vi "Dialog Box - One Button.vi"(4 "Display On Error (True)":bool=TRUE, 6 "Display (True)":bool=TRUE, 7 "Timeout (Seconds)":i16=-1, 8 "error in (no error)":errorcluster, 11 "Text":string) -> (0 "error out":errorcluster)   [LabVIEW 2011]
doc: "Displays a simple one button dialog box.\n\nA timeout can be set. If no timeout is defined then the dialog will wait forever.\n\nIf \"Display\" input is False then no dialog will be displayed.\nIf \"Display on Error\" is False and an Error has occured then the dialog will not be display.\n\nThis dialog box will increase in size if required depending on the supplied text."
panel:
  in  "OK Button":bool
  out "String":string
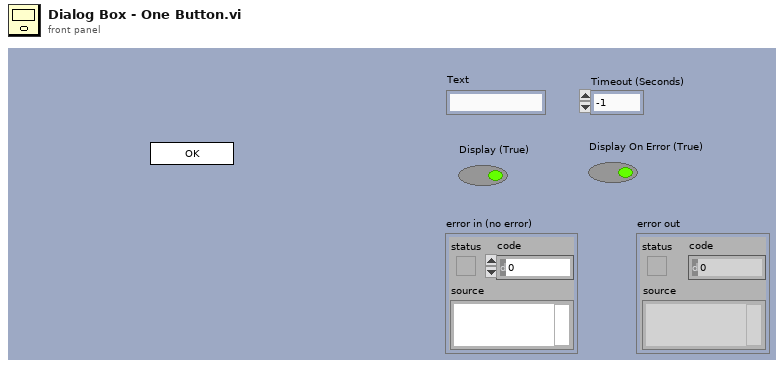
[diagram p1: front panel]
types:
  T1 = enum32{"Invalid", "Default", "Floating", "Floating/Auto-Hide", "Modal"}
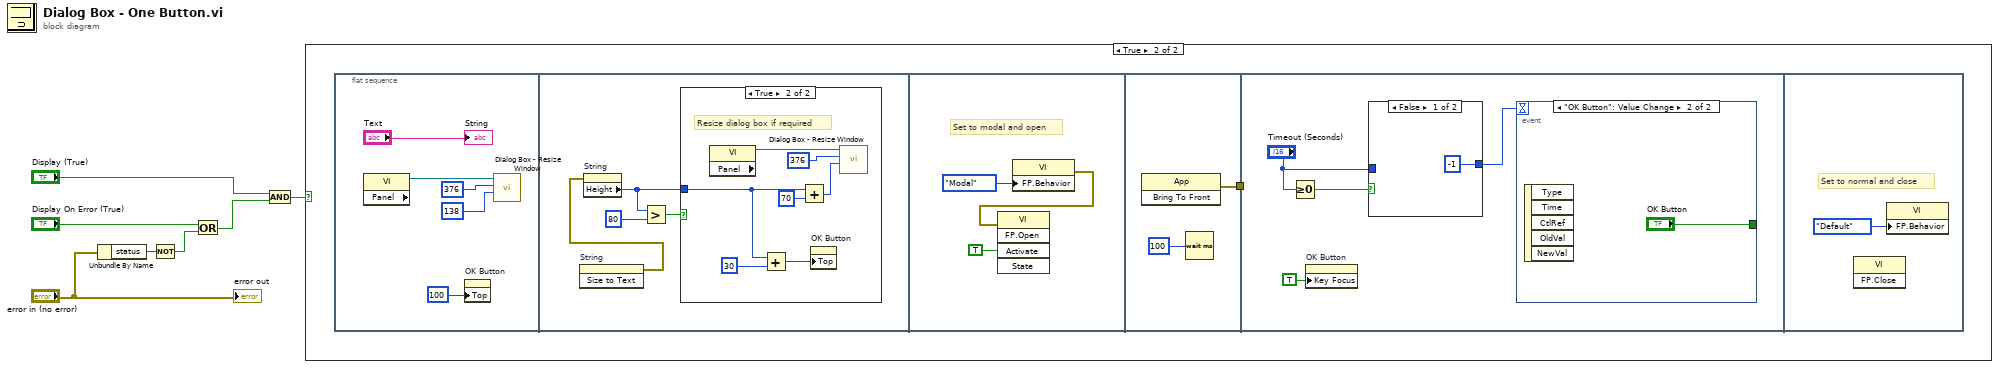
[diagram p0: block diagram]
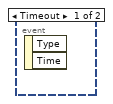
[diagram p4: hidden frame]
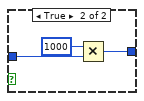
[diagram p5: hidden frame]
diagram:
  n1 = Unbundle By Name("error in (no error)") -> ("status"=w2:bool)
  n2 = Not(x=w2) -> (.not. x?=w1:bool)
  n3 = Or(x="Display On Error (True)", y=w1) -> (x .or. y?=w4:bool)
  n4 = And(x="Display (True)", y=w4) -> (x .and. y?=w5:bool)
  n5 = case shown="True" w5 {
    frame False {
    }
    frame True {
      n6 = flat-sequence {
        tunnel: [w29] -> w8
        tunnel: w8 -> [_]
        frame #0 {
          n7 = property class="VI" props=["Panel"]() -> (reference out=w12:refnum<vi>)  [unwired: 2 in, 2 out]
          n8 = property on="OK Button" class="Bool"("Top"=100 ("Position:Top")) -> ()  [unwired: 2 in, 2 out]
          n9 = call "Dialog Box - Resize Window.vi"("Height"=i16 138, "Width"=i16 376, "reference"=w12) -> ()  [unwired: 8 in, 1 out]
          "String" <- "Text"
        }
        frame #1 {
          n10 = invoke on="String" class="Str" method="Size to Text"() -> (error out=w14:errorcluster)  [unwired: 3 in, 2 out]
          n11 = property on="String" class="Str"(error in=w14) -> ("Height"=w15:u32)  [unwired: 1 in, 2 out]
          n12 = Greater?(x=w15, y=u32 80) -> (0:w16:bool)
          n13 = case shown="True" w16 {
            tunnel: w15 -> [_ w20]
            frame False {
            }
            frame True {
              # "Resize dialog box if required"
              n14 = property class="VI" props=["Panel"]() -> (reference out=w24:refnum<vi>)  [unwired: 2 in, 2 out]
              n15 = Add(x=w20, y=u32 30) -> (x+y=w19:u32)
              n16 = Add(x=w20, y=u32 70) -> (x+y=w22:u32)
              n17 = property on="OK Button" class="Bool"("Top"=w19) -> ()  [unwired: 2 in, 2 out]
              n18 = call "Dialog Box - Resize Window.vi"("Height"=w22, "Width"=i16 376, "reference"=w24) -> ()  [unwired: 8 in, 1 out]
            }
          }
        }
        frame #2 {
          # "Set to modal and open"
          n19 = property class="VI"("FP.Behavior"=T1."Modal" ("Front Panel Window:Behavior")) -> (error out=w25:errorcluster)  [unwired: 2 in, 1 out]
          n20 = invoke class="VI" method="FP.Open"(error in=w25, "Activate"=TRUE ("Activate?")) -> ()  [unwired: 3 in, 5 out]
        }
        frame #3 {
          n21 = invoke class="App" method="Bring To Front"() -> (error out=w29:errorcluster)  [unwired: 3 in, 2 out]
          n22 = Wait (ms)(milliseconds to wait=u32 100) -> ()  [unwired: 1 out]
        }
        frame #4 {
          n23 = Greater Or Equal To 0?(x="Timeout (Seconds)") -> (x >= 0?=w33:bool)
          n24 = property on="OK Button" class="Bool"("Key Focus"=TRUE) -> ()  [unwired: 2 in, 2 out]
          n25 = case shown="False" w33 {
            tunnel: "Timeout (Seconds)" -> [_ w38]
            tunnel: [i16 -1 w36] -> w31
            frame False {
            }
            frame True {
              n26 = Multiply(x=i16 1000, y=w38) -> (x*y=w36:i16)
            }
          }
          n27 = event shown="[1] \"OK Button\": Value Change" {
            selector: _ -> [_ _]
            dyn-events: _ -> [_ _]
            timeout: w31 -> [_ _]
            tunnel: [_ "OK Button"] -> _
            event Timeout {
              n28 = event-data() -> ()  [unwired: 1 in, 2 out]
            }
            event "OK Button": Value Change {
              n29 = event-data() -> ()  [unwired: 1 in, 5 out]
            }
          }
        }
        frame #5 {
          # "Set to normal and close"
          n30 = invoke class="VI" method="FP.Close"() -> ()  [unwired: 3 in, 3 out]
          n31 = property class="VI"("FP.Behavior"=T1."Default" ("Front Panel Window:Behavior")) -> ()  [unwired: 2 in, 2 out]
        }
      }
    }
  }
  "error out" <- "error in (no error)"
